vi "WSP2_BackCheck_Serial.vi"(0 "serialNumber":string, 1 "stationName":string) -> (2 "Status":i8, 3 "ReplyTracMex":string, 4 "error out":errorcluster)   [LabVIEW 2023]
uses:
  C:/Elatch-Bench-Test/WSConnector/WSConnector.dll
  WSConnector/WSConnector.dll
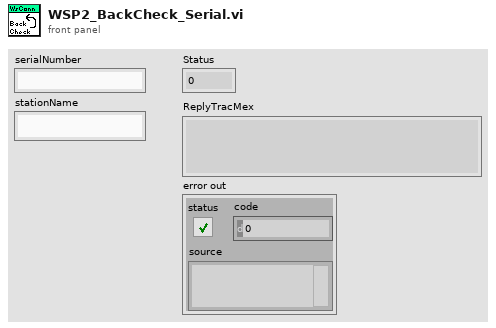
[diagram p1: front panel]
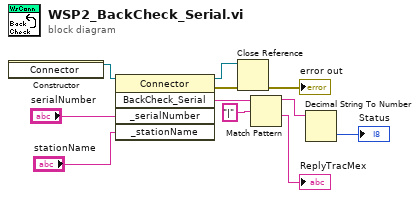
[diagram p0: block diagram]
diagram:
  n1 = constructor class="Connector"() -> (reference out=w11:refnum<k24>)  [unwired: 3 in, 2 out]
  n2 = invoke class="Connector" method="BackCheck_Serial"(reference=w11, "_serialNumber"="serialNumber", "_stationName"="stationName") -> (reference out=w2:refnum<k24>, error out=w3:errorcluster, "BackCheck_Serial"=w5:string)  [unwired: 2 in, 2 out]
  n3 = Close Reference(reference=w2, error in (no error)=w3) -> (error out=→"error out":errorcluster)
  n4 = Match Pattern(string=w5, regular expression="|") -> (before substring=w7:string, after substring=→"ReplyTracMex":string)  [unwired: 1 in, 2 out]
  n5 = Decimal String To Number(string=w7) -> (number=→"Status":i32)  [unwired: 2 in, 1 out]
